vi "CallWeb.vi"() -> ()   [LabVIEW 2014]
uses:
  <vilib>/addons/database/Auxilliary.llb/DB Tools Format Datetime String (Time Stamp).vi
  <vilib>/httpClient/LabVIEWHTTPClient.lvlib
  <vilib>/addons/database/NI_Database_API.lvlib
panel:
  in  "Longitud":string="-66.88\n"
  in  "Latitud":string="10.41"
  in  "Fecha final":timestamp format="%<%Y/%m/%d>T"
  in  "Fecha inicial":timestamp format="%<%Y/%m/%d>T"
  out "body":string
  out "headers":string
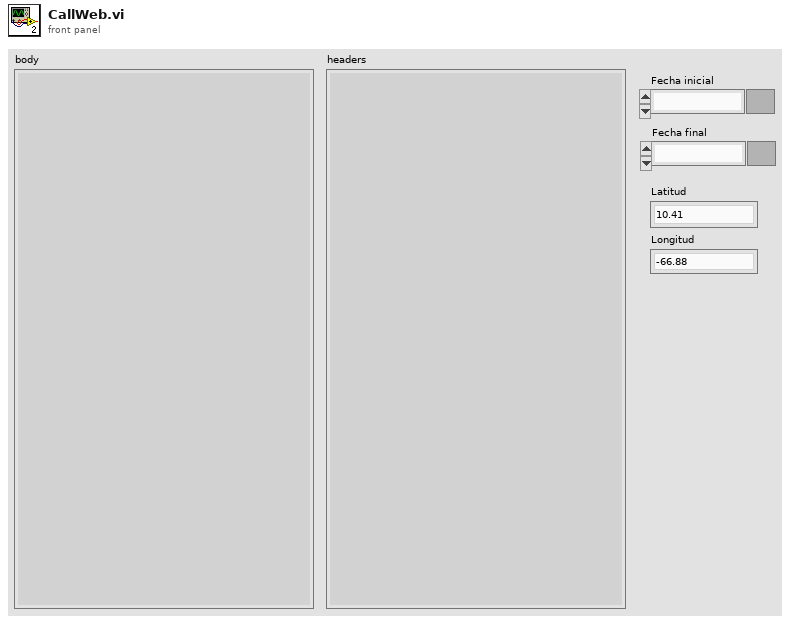
[diagram p1: front panel]
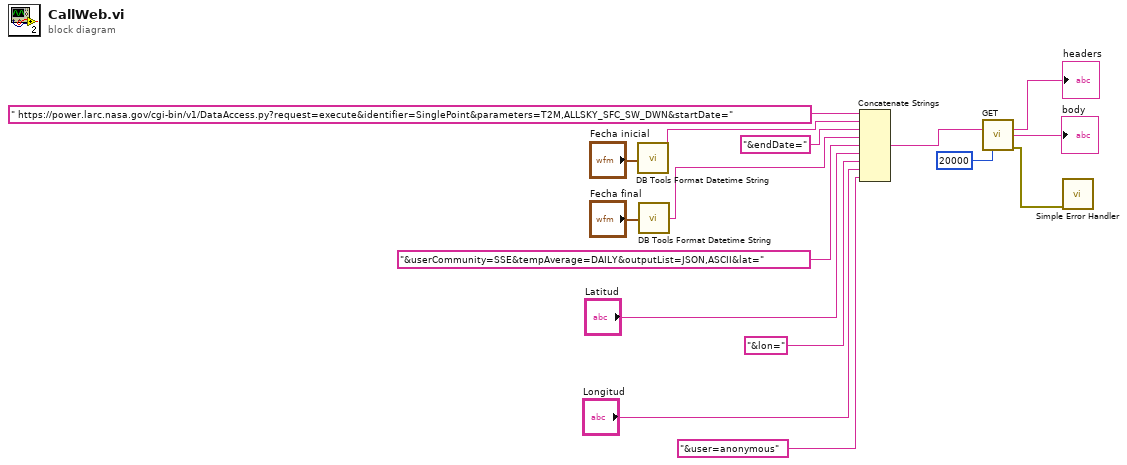
[diagram p0: block diagram]
diagram:
  n1 = call-poly <vilib>:"DB Tools Format Datetime String.vi"("time stamp"="Fecha inicial") -> ("date/time string"=w11:string)
  n2 = call-poly <vilib>:"DB Tools Format Datetime String.vi"("time stamp"="Fecha final") -> ("date/time string"=w5:string)
  n3 = Concatenate Strings(" https://power.larc.nasa.gov/cgi-bin/v1/DataAccess.py?request=execute&identifier=SinglePoint&parameters=T2M,ALLSKY_SFC_SW_DWN&startDate=", w11, "&endDate=", w5, "&userCommunity=SSE&tempAverage=DAILY&outputList=JSON,ASCII&lat=" ("url"), "Latitud", "&lon=" ("url"), "Longitud", "&user=anonymous" ("url")) -> (w8:string)
  n4 = call <vilib>:"GET.vi"("url"=w8, "timeout (10000)"=20000) -> ("headers"=→"headers":string, "body"=→"body":string, "error out"=w13:errorcluster)  [unwired: 10 in, 1 out]
  n5 = call <vilib>:"Simple Error Handler.vi"("error in (no error)"=w13) -> ()  [unwired: 4 in, 5 out]
